vi "listen connection LV15.vi"(8 "Bool Refnum":refnum<vi>, 10 "service name":string="192.168.1.10") -> (2 "Boolean 3":bool, 3 "data out":string)   [LabVIEW 2015]
uses:
  Galobal variable_TI.vi
panel:
  out "String":string
  out "Coordinate 3":string
  out "Numeric 2":i32
  out "error out 3":errorcluster
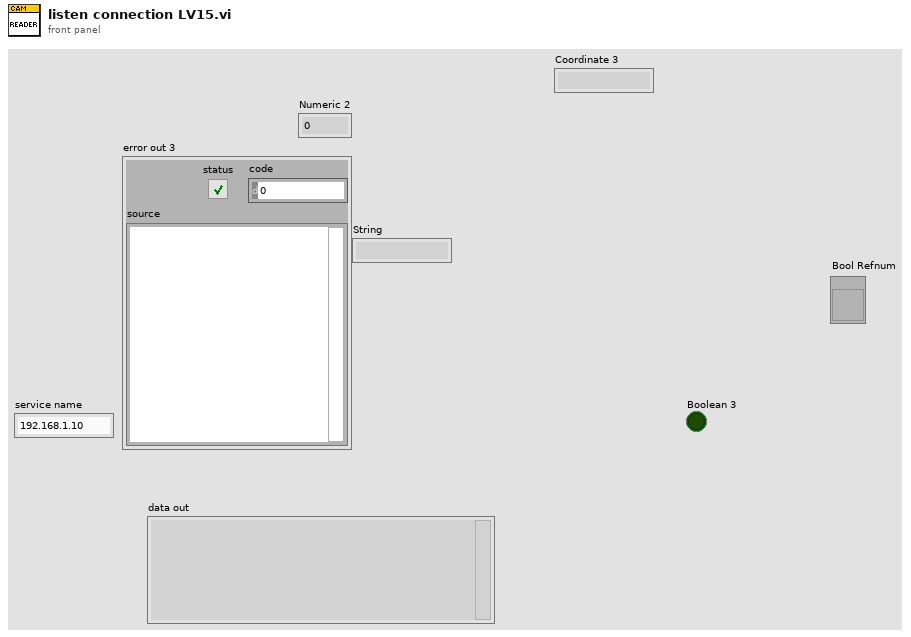
[diagram p1: front panel]
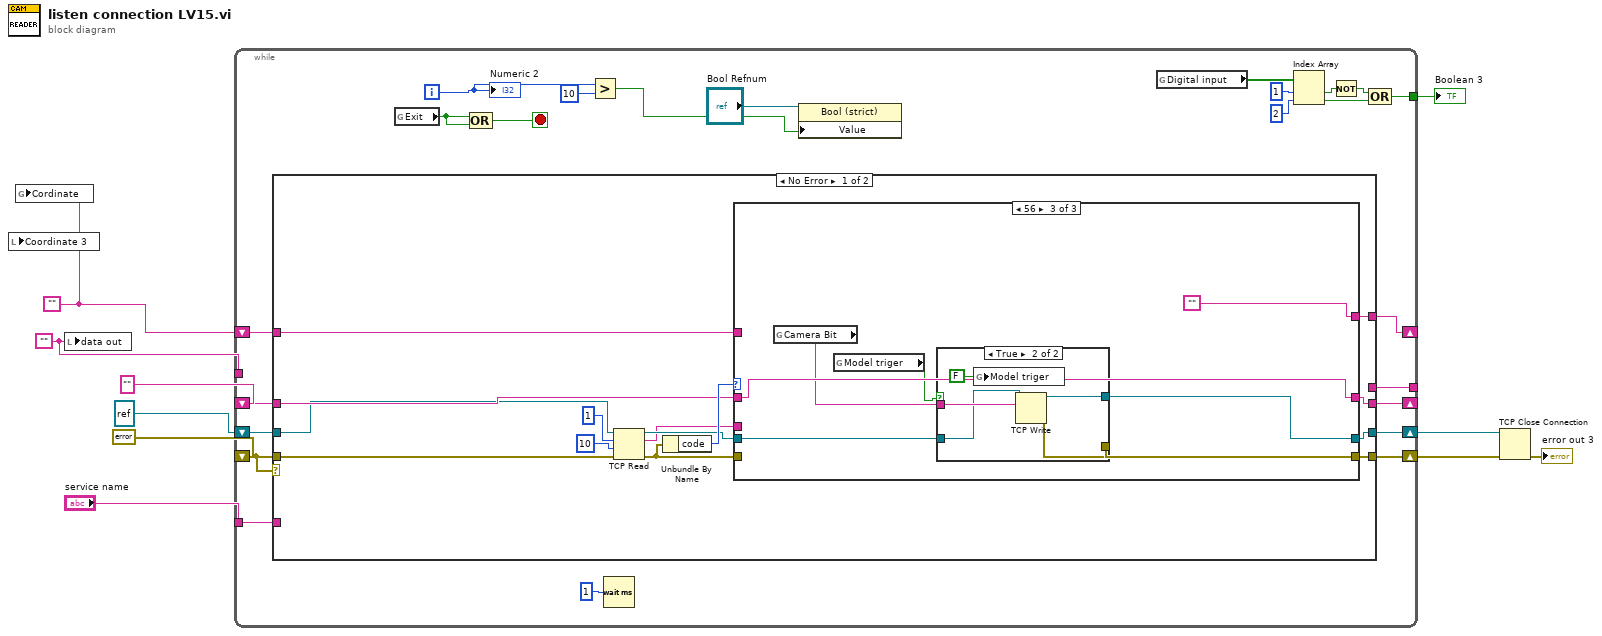
[diagram p0: block diagram]
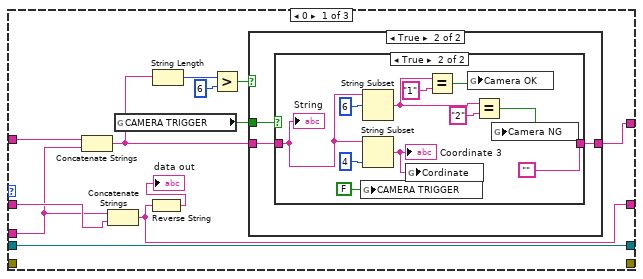
[diagram p2: hidden frame]
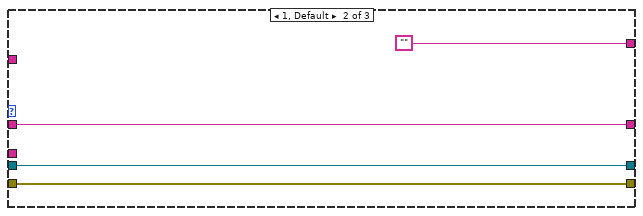
[diagram p5: hidden frame]
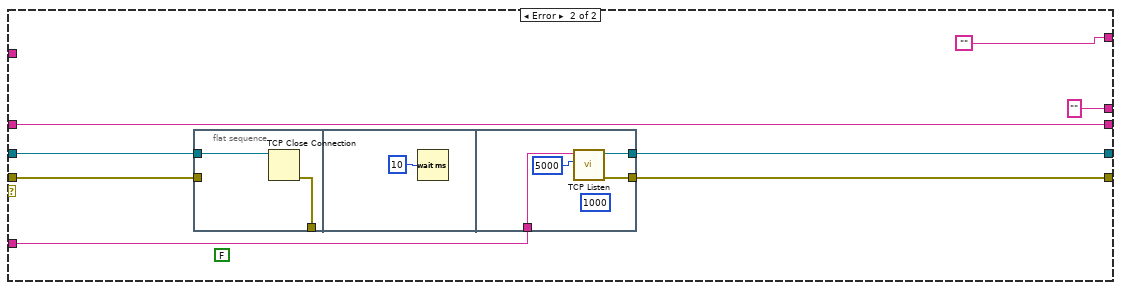
[diagram p7: hidden frame]
diagram:
  w1 = ""
  w2 = ""
  n1 = local write "Coordinate 3"(w1) -> ()
  n2 = global write "Galobal variable_TI.vi" "Cordinate"(w1) -> ()
  n3 = local write "data out"(w2) -> ()
  n4 = while {
    tunnel: [w32] -> _
    shift-right: [w34] -> w10
    shift-left: refnum<k5> refnum ("connection ID") -> [w31]
    shift-right: [w33] -> w9
    shift-left: errorcluster {"status"=FALSE, "code"=0, "source"=""} ("error out") -> [w30]
    tunnel: "service name" -> [w29]
    shift-right: [w19] -> _
    shift-left: "" -> [w28]
    tunnel: [w18] -> w3
    tunnel: w2 -> [_]
    shift-right: [w15] -> _
    shift-left: w1 -> [w16]
    i -> [w14]
    stop <- w26 stop-if-true
    n5 = case shown="No Error" w30 {
      tunnel: [w45 w97] -> w34
      tunnel: [w44 w96] -> w33
      tunnel: [_ "" ("data out")] -> w32
      tunnel: w31 -> [w36 w101]
      tunnel: w30 -> [w35 w100]
      tunnel: w29 -> [_ w99]
      tunnel: [w39 w98] -> w19
      tunnel: w28 -> [w41 w98]
      tunnel: w16 -> [w38 _]
      tunnel: [w37 ""] -> w15
      frame No Error {
        n6 = TCP Read(connection ID=w36, bytes to read=1, error in (no error)=w35, 9:10 ("timeout ms (25000)")) -> (connection ID out=w46:refnum<k5>, data out=w42:string, error out=w43:errorcluster)  [unwired: 1 in]
        n7 = Unbundle By Name(w43) -> ("code"=w47:i32)
        n8 = case shown="56" w47 {
          tunnel: w46 -> [w60 w79 w82]
          tunnel: [w60 w79 w84] -> w45
          tunnel: [_ w80 w83] -> w44
          tunnel: w43 -> [_ w80 _]
          tunnel: w42 -> [w51 _ _]
          tunnel: [w53 w78 w87] -> w39
          tunnel: w41 -> [w54 w78 w87]
          tunnel: w38 -> [w52 _ _]
          tunnel: [w50 "" ""] -> w37
          frame 0 {
            n9 = Concatenate Strings(w52, w51) -> (w49:string)
            n10 = Concatenate Strings(w51, w54) -> (w53:string)
            n11 = global read "Galobal variable_TI.vi" "CAMERA TRIGGER"() -> (w57:bool)
            n12 = Reverse String(1:w53) -> (0:→"data out":string)
            n13 = String Length(string=w49) -> (length=w59:i32)
            n14 = Greater?(x=w59, y=6) -> (0:w58:bool)
            n15 = case shown="True" w58 {
              tunnel: w57 -> [_ w64]
              tunnel: w49 -> [w61 w63]
              tunnel: [w61 w62] -> w50
              frame False {
              }
              frame True {
                n16 = case shown="True" w64 {
                  tunnel: w63 -> [w65 w67]
                  tunnel: [w65 ""] -> w62
                  frame False {
                  }
                  frame True {
                    n17 = global write "Galobal variable_TI.vi" "CAMERA TRIGGER"(FALSE ("CAMERA TRIGGER")) -> ()
                    n18 = String Subset(string=w67, offset (0)=6) -> (substring=w70:string)  [unwired: 1 in]
                    n19 = String Subset(string=w67, length (rest)=4 ("length (rest)")) -> (substring=w76:string)  [unwired: 1 in]
                    "Coordinate 3" <- w76
                    n20 = global write "Galobal variable_TI.vi" "Cordinate"(w76) -> ()
                    n21 = Equal?(x=w70, y="1") -> (x = y?=w69:bool)
                    n22 = global write "Galobal variable_TI.vi" "Camera OK"(w69) -> ()
                    n23 = Equal?(x=w70, y="2") -> (x = y?=w68:bool)
                    n24 = global write "Galobal variable_TI.vi" "Camera NG"(w68) -> ()
                    "String" <- w67
                  }
                }
              }
            }
          }
          frame 1, Default {
          }
          frame 56 {
            n25 = global read "Galobal variable_TI.vi" "Camera Bit"() -> (w85:string)
            n26 = global read "Galobal variable_TI.vi" "Model triger"() -> (w81:bool)
            n27 = case shown="True" w81 {
              tunnel: w85 -> [_ w93]
              tunnel: [w88 w92] -> w84
              tunnel: [_ w91] -> w83
              tunnel: w82 -> [w88 w90]
              frame False {
              }
              frame True {
                n28 = global write "Galobal variable_TI.vi" "Model triger"(FALSE ("Model triger")) -> ()
                n29 = TCP Write(connection ID=w90, data in=w93) -> (connection ID out=w92:refnum<k5>, error out=w91:errorcluster)  [unwired: 2 in, 1 out]
              }
            }
          }
        }
      }
      frame Error {
        (unwired) FALSE
        n30 = flat-sequence {
          tunnel: w101 -> [w103]
          tunnel: w100 -> [_]
          tunnel: [w102] -> _
          tunnel: w99 -> [w107]
          tunnel: [w106] -> w97
          tunnel: [w105] -> w96
          frame #0 {
            n31 = TCP Close Connection(connection ID=w103) -> (error out=w102:errorcluster)  [unwired: 2 in, 1 out]
          }
          frame #1 {
            n32 = Wait (ms)(milliseconds to wait=u32 10) -> ()  [unwired: 1 out]
          }
          frame #2 {
            (unwired) 1000 ("timeout ms (wait forever: -1)")
            n33 = call <vilib>:"TCP Listen.vi"("port"=u16 5000, "service name"=w107) -> ("error out"=w105:errorcluster, "connection ID"=w106:refnum<k5>)  [unwired: 5 in, 3 out]
          }
        }
      }
    }
    n34 = global read "Galobal variable_TI.vi" "Exit"() -> (w17:bool)
    n35 = Compound Arithmetic op=OR(w17, w17) -> (w26:bool)
    n36 = Greater?(x=w14, y=10) -> (0:w11:bool)
    n37 = Wait (ms)(milliseconds to wait=u32 1) -> ()  [unwired: 1 out]
    n38 = property class="Bool (strict)"(reference="Bool Refnum", "Value"=w11) -> ()  [unwired: 1 in, 2 out]
    n39 = global read "Galobal variable_TI.vi" "Digital input"() -> (w25:bool[])
    n40 = Index Array(array=w25, index #1=1 ("index"), index #2=2 ("index")) -> (element #1=w22:bool, element #2=w20:bool)
    n41 = Not(x=w22) -> (.not. x?=w21:bool)
    n42 = Compound Arithmetic op=OR(w21, w20) -> (w18:bool)
    "Numeric 2" <- w14
  }
  "Boolean 3" <- w3
  n43 = TCP Close Connection(connection ID=w10, error in (no error)=w9) -> (error out=→"error out 3":errorcluster)  [unwired: 1 in, 1 out]
